vi "System Monitor Initialization VI.vi"(8 "error in (no error)":errorcluster, 10 "Custom XML":string, 11 "Device Item Ref in":T1 format="%.0x") -> (0 "error out":errorcluster, 3 "Device Item Ref out":T1 format="%.0x")   [LabVIEW 2011, in "System Monitor Custom Device.lvlib"]
uses:
  System Monitor Custom Device.lvlib
  <vilib>/NI Veristand/Custom Device API/Custom Device Item Ref.ctl
  <vilib>/NI Veristand/Custom Device API/Custom Device Channel Type.ctl
  <vilib>/NI Veristand/Custom Device API/Custom Device Channel.ctl
  <vilib>/NI Veristand/Custom Device API/Set Item Property (I32).vi
  <vilib>/NI Veristand/Custom Device API/Custom Device API.lvlib
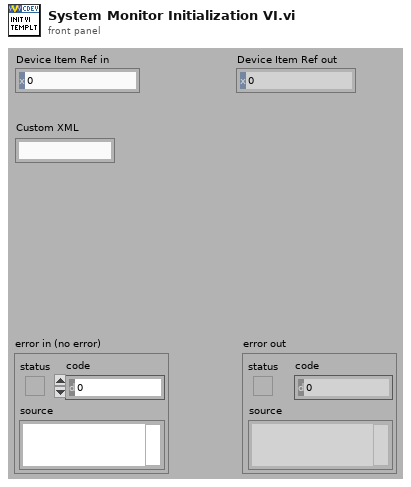
[diagram p1: front panel]
types:
  T1 = typedef "Custom Device API.lvlib/Custom Device Item Ref.ctl" = u64
  T2 = typedef "Custom Device API.lvlib/Custom Device Channel Type.ctl" = enum16{"Input", "Output"}
  T3 = typedef "Custom Device API.lvlib/Custom Device Channel.ctl" = cluster{"Type":T2, "Units":string, "Default Value":dbl, "Faultable":bool, "Scalable":bool}
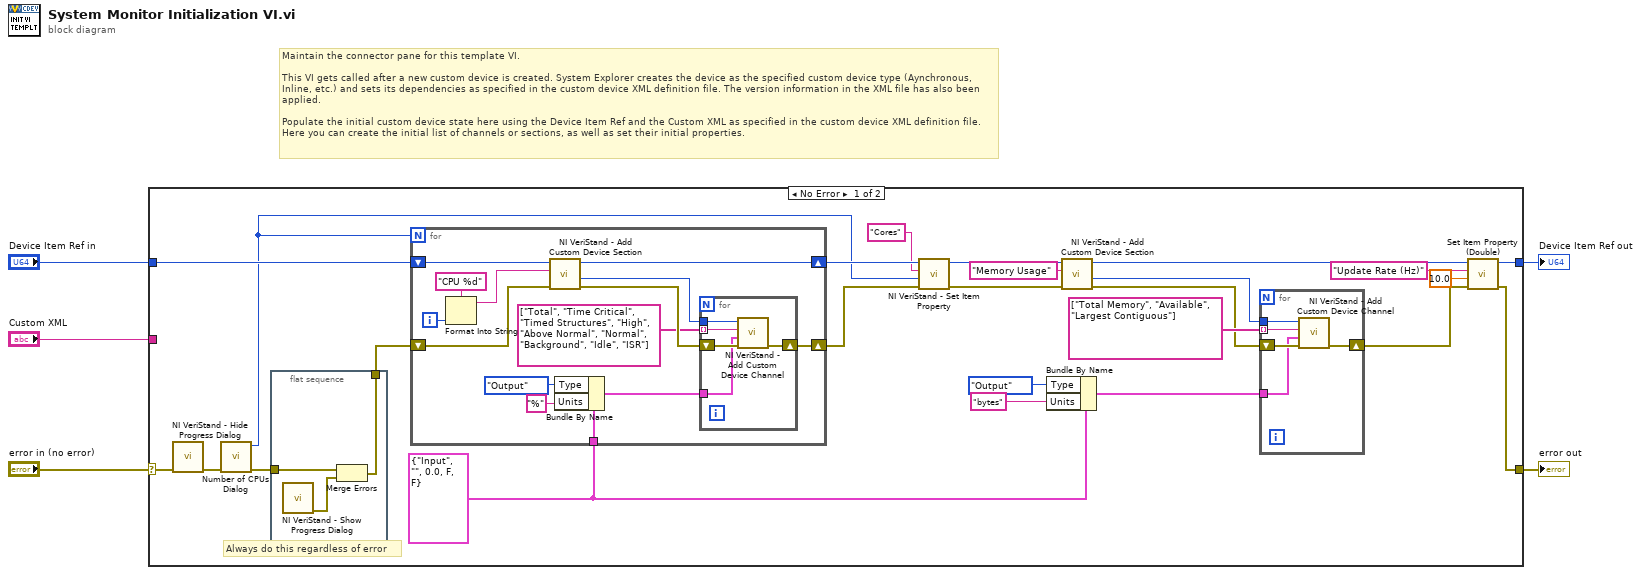
[diagram p0: block diagram]
diagram:
  # "Maintain the connector pane for this template VI.\n\nThis VI gets called after a new custom device is created. System Explorer creates the device as the specified custom device type (Aynchronous, Inline, etc.) and sets its dependencies as specified in the custom device XML definition file. The version information in the XML file has also been applied.\n\nPopulate the initial custom device state here using the Device Item Ref and the Custom XML as specified in the custom device XML definition file. Here you can create the initial list of channels or sections, as well as set their initial properties."
  n1 = case shown="No Error" "error in (no error)" {
    selector: "error in (no error)" -> [w15 w59]
    tunnel: [w17 w59] -> w5
    tunnel: [w16 w58] -> w3
    tunnel: "Device Item Ref in" -> [w18 w58]
    tunnel: "Custom XML" -> [_ _]
    frame No Error {
      w24 = T3 {"Type"=enum."Input", "Units"="", "Default Value"=0.0, "Faultable"=FALSE, "Scalable"=FALSE} ("Channel")
      # "Always do this regardless of error"
      n2 = call <vilib>:"NI VeriStand - Hide Progress Dialog.vi"("error in (no error)"=w15) -> ("error out"=w14:errorcluster)  [unwired: 10 in]
      n3 = call "Number of CPUs Dialog.vi"("error in (no error)"=w14) -> ("error out"=w13:errorcluster, "CPU_Cores"=w6:i32)  [unwired: 9 in]
      n4 = flat-sequence {
        tunnel: w13 -> [w33]
        tunnel: [w31] -> w12
        frame #0 {
          n5 = call <vilib>:"NI VeriStand - Show Progress Dialog.vi"() -> ("error out"=w32:errorcluster)  [unwired: 11 in]
          n6 = Merge Errors(w33, w32) -> (w31:errorcluster)
        }
      }
      n7 = for {
        N: w6 -> [_]
        shift-right: [w50] -> w11
        shift-left: w18 -> [w52]
        shift-right: [w40] -> w8
        shift-left: w12 -> [w46]
        tunnel: w24 -> [w39]
        i -> [w48]
        n8 = Format Into String(format string="CPU %d" ("Section Name"), w48) -> (resulting string=w47:string)  [unwired: 2 in, 1 out]
        n9 = call <vilib>:"NI VeriStand - Add Custom Device Section.vi"("error in (no error)"=w46, "Section Name"=w47, "Parent Ref in"=w52) -> ("error out"=w45:errorcluster, "Section Ptr"=w51:T1, "Parent Ref out"=w50:T1)  [unwired: 5 in, 1 out]
        n10 = Bundle By Name(cluster=w39, "Type"=Custom_Device_Channel_Type."Output", "Units"="%") -> (w41:T3)
        n11 = for {
          tunnel: w51 -> [w57]
          shift-right: [w55] -> w40
          shift-left: w45 -> [w56]
          tunnel: string[] ["Total", "Time Critical", "Timed Structures", "High", "Above Normal", "Normal", "Background", "Idle", "ISR"] -> [w54] mode=indexing
          tunnel: w41 -> [w53]
          n12 = call <vilib>:"NI VeriStand - Add Custom Device Channel.vi"("error in (no error)"=w56, "Channel"=w53, "Channel Name"=w54, "Parent Ref in"=w57) -> ("error out"=w55:errorcluster)  [unwired: 4 in, 3 out]
        }
      }
      n13 = call-poly <vilib>:"NI VeriStand - Set Item Property.vi"("error in (no error)"=w8, "Value"=w6, "Property Name"="Cores", "Item Ref in"=w11) -> ("error out"=w9:errorcluster, "Item Ref out"=w10:T1)  [unwired: 5 in, 1 out]
      n14 = Bundle By Name(cluster=w24, "Type"=Custom_Device_Channel_Type."Output", "Units"="bytes") -> (w26:T3)
      n15 = call <vilib>:"NI VeriStand - Add Custom Device Section.vi"("error in (no error)"=w9, "Section Name"="Memory Usage", "Parent Ref in"=w10) -> ("error out"=w20:errorcluster, "Section Ptr"=w21:T1, "Parent Ref out"=w27:T1)  [unwired: 5 in, 1 out]
      n16 = for {
        tunnel: w21 -> [w37]
        shift-right: [w36] -> w28
        shift-left: w20 -> [w38]
        tunnel: string[] ["Total Memory", "Available", "Largest Contiguous"] -> [w35] mode=indexing
        tunnel: w26 -> [w34]
        n17 = call <vilib>:"NI VeriStand - Add Custom Device Channel.vi"("error in (no error)"=w38, "Channel"=w34, "Channel Name"=w35, "Parent Ref in"=w37) -> ("error out"=w36:errorcluster)  [unwired: 4 in, 3 out]
      }
      n18 = call <vilib>:"Set Item Property (Double).vi"("error in (no error)"=w28, "Value"=10.0, "Property Name"="Update Rate (Hz)", "Item Ref in"=w27) -> ("error out"=w17:errorcluster, "Item Ref out"=w16:T1)  [unwired: 5 in, 1 out]
    }
    frame Error {
    }
  }
  "error out" <- w5
  "Device Item Ref out" <- w3
